vi "Create.vi"(8 "error in (no error)":errorcluster, 11 "Server in":refnum<class "Server.lvclass">) -> (0 "error out":errorcluster, 3 "Server out":refnum<class "Server.lvclass">)   [LabVIEW 2020, in "Server.lvlib" / "Server.lvclass"]
uses:
  Server.lvclass
  Server.lvclass/Server.ctl
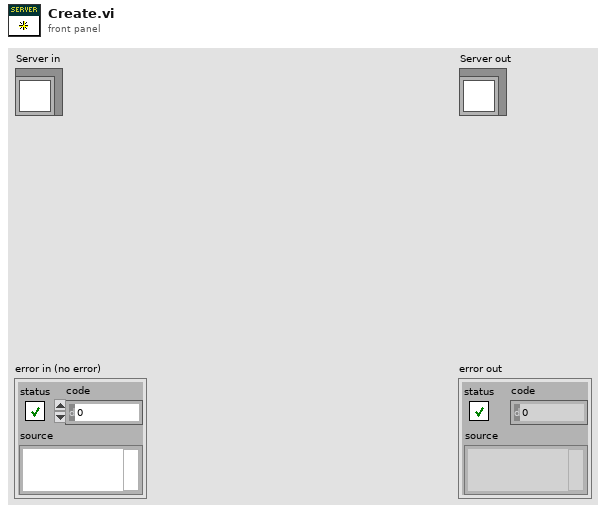
[diagram p1: front panel]
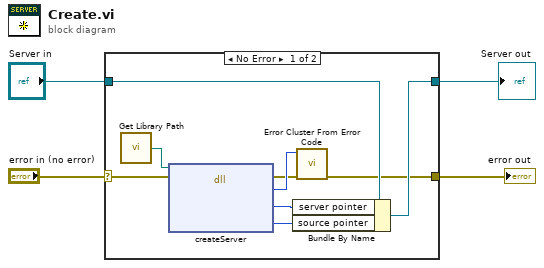
[diagram p0: block diagram]
diagram:
  n1 = case shown="No Error" "error in (no error)" {
    selector: "error in (no error)" -> [w11 w15]
    tunnel: [w8 w15] -> w2
    tunnel: [w12 w14] -> w3
    tunnel: "Server in" -> [w13 w14]
    frame No Error {
      n2 = call "Get Library Path.vi"() -> ("Path"=w6:path)  [unwired: 1 in]
      n3 = dll-call lib="?" fn="createServer"(path in=w6, error in=w11) -> (error out=w9:errorcluster, "ret code"=w10:i32, "server"=w7:i64, "source"=w5:i64)  [unwired: 3 in, 1 out]
      n4 = Bundle By Name(cluster=w13, "server pointer"=w7, "source pointer"=w5) -> (w12:refnum<class "Server.lvclass">)
      n5 = call <vilib>:"Error Cluster From Error Code.vi"("error in (no error)"=w9, "error code (0)"=w10) -> ("error out"=w8:errorcluster)  [unwired: 7 in]
    }
    frame Error {
    }
  }
  "error out" <- w2
  "Server out" <- w3
